vi "dfd_TF to Lattice MA.vi"(10 "denominator":dbl[](array[numeric]) format="%.2f", 11 "numerator":dbl[](array[numeric]) format="%.2f") -> (0 "fail?":bool, 1 "gain":dbl format="%.2f", 2 "k [1~M]":dbl[](array[numeric]) format="%.2f")   [LabVIEW 2017, in "NI_DigFilterLicensed.lvlib"]
uses:
  <vilib>/addons/Digital Filter Design/NI_DigFilterLicensed.lvlib
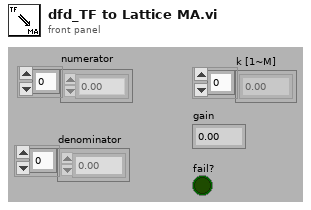
[diagram p1: front panel]
types:
  T1 = enum16{"Basic Section", "One Multiplier Section", "Normalized Section"}
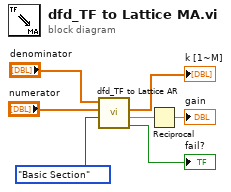
[diagram p0: block diagram]
diagram:
  n1 = call <vilib>:"dfd_TF to Lattice AR.vi"("section type"=T1."Basic Section", "denominator"="numerator", "numerator"="denominator") -> ("fail?"=→"fail?":bool, "gain"=w5:dbl, "k [1~M]"=→"k [1~M]":dbl[])  [unwired: 6 out]
  n2 = Reciprocal(x=w5) -> (1/x=→"gain":dbl)
